vi "email_Donnee.vi"(8 "entrée d'erreur (pas d'erreur)":errorcluster, 11 "tableau_config":string[](array[string])) -> (0 "sortie d'erreur":errorcluster)   [LabVIEW 2020]
panel:
  out "trimmed string":string
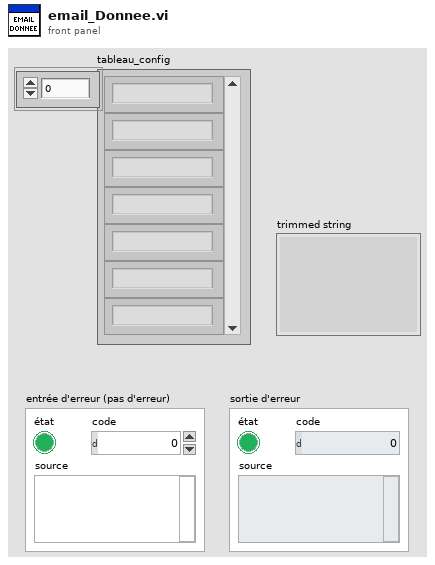
[diagram p1: front panel]
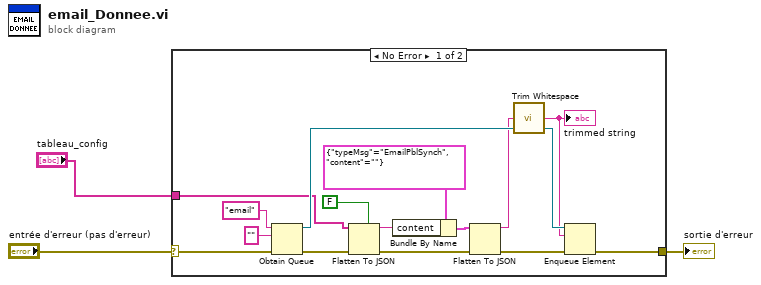
[diagram p0: block diagram]
diagram:
  n1 = case shown="No Error" "entrée d'erreur (pas d'erreur)" {
    selector: "entrée d'erreur (pas d'erreur)" -> [w17 w19]
    tunnel: [w14 w19] -> w2
    tunnel: "tableau_config" -> [w4 _]
    frame No Error {
      n2 = Obtain Queue(name (unnamed)="email" ("nom (aucun)"), element data type="" ("nom (aucun)"), error in (no error)=w17) -> (queue out=w15:refnum<queue>, error out=w16:errorcluster)  [unwired: 2 in, 1 out]
      n3 = Flatten To JSON(enable LabVIEW extensions? (T)=FALSE ("activer les extensions LabVIEW ? (V)"), anything=w4, error in (no error)=w16) -> (JSON string=w11:string, 11:w6:errorcluster)
      n4 = Bundle By Name(cluster=cluster{"typeMsg":string, "content":string} {"typeMsg"="EmailPblSynch", "content"=""}, "content"=w11) -> (w10:cluster{"typeMsg":string, "content":string})
      n5 = Flatten To JSON(anything=w10, error in (no error)=w6) -> (JSON string=w9:string, 11:w5:errorcluster)  [unwired: 1 in]
      n6 = call <vilib>:"Trim Whitespace.vi"("string"=w9) -> ("trimmed string"=w13:string)  [unwired: 1 in]
      "trimmed string" <- w13
      n7 = Enqueue Element(queue=w15, element=w13, error in (no error)=w5) -> (error out=w14:errorcluster)  [unwired: 1 in, 2 out]
    }
    frame Error {
    }
  }
  "sortie d'erreur" <- w2
